vi "Drag & Drop New.vi"   [LabVIEW 2015]
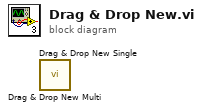
[diagram p0: block diagram]
diagram:
  n1 = call "Drag & Drop New Multi.vi"() -> ()  [unwired: 9 in, 2 out]
  n2 = call "Drag & Drop New Single.vi"() -> ()  [unwired: 9 in, 2 out]
